vi "Update History Messages.vi"(8 "error in (no error)":errorcluster, 10 "Message":variant, 11 "Telegram Class in":refnum<class "Telegram Class.lvclass">) -> (0 "error out":errorcluster, 3 "Telegram Class out":refnum<class "Telegram Class.lvclass">)   [LabVIEW 2015, in "Telegram Library.lvlib" / "Telegram Class.lvclass"]
doc: "Created IvanLis by LabVIEW Portal\nProfile: http://labviewportal.org/memberlist.php?mode=viewprofile&u=987\neMail: IvanLisanov@gMail.com\nTelegram: https://t.me/IvanLis"
uses:
  Telegram Class.lvclass
  JSON Library/TypeDef/Message Text.ctl
  Telegram Class.lvclass/Telegram Class.ctl
  TypeDef/Message.ctl
  JSON Library/JSON Library.lvlib
  Telegram Library.lvlib
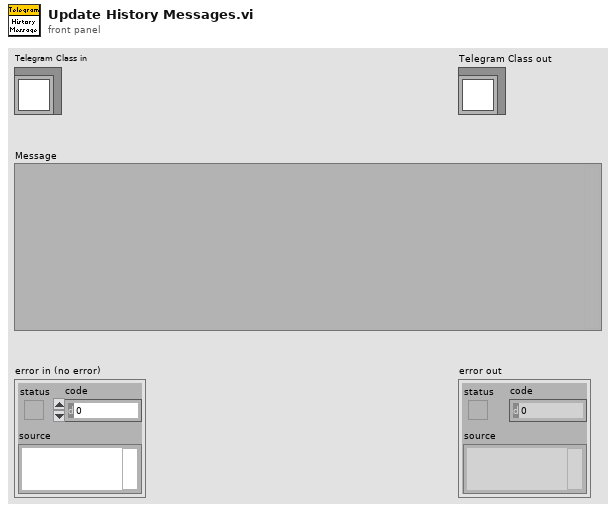
[diagram p1: front panel]
types:
  T1 = typedef "JSON Library.lvlib/Message Text.ctl" = cluster{"@type":string, "id":i64, "sender_id":cluster{"@type":string, "user_id":i64}, "chat_id":i64, "date":i64, "content":cluster{"@type":string, "text":cluster{"@type":string, "text":string}}}
  T2 = typedef "Telegram Library.lvlib/Message.ctl" = cluster{"id":i64, "chat_id":i64, "sender_user_id":i64, "date UTC":timestamp, "content_text":string}
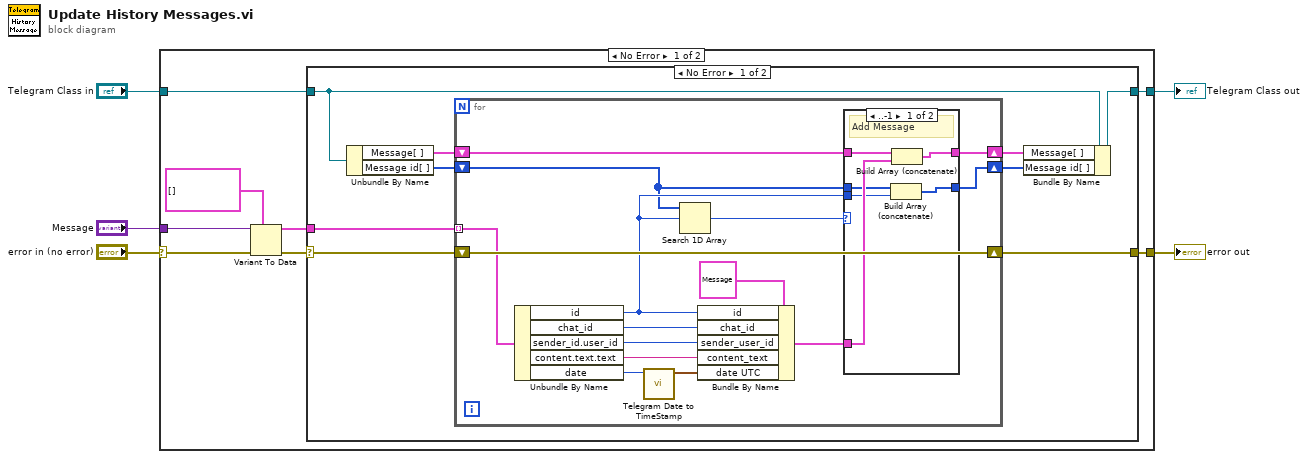
[diagram p0: block diagram]
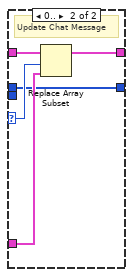
[diagram p2: hidden frame]
diagram:
  n1 = case shown="No Error" "error in (no error)" {
    selector: "error in (no error)" -> [w13 w52]
    tunnel: [w7 w52] -> w4
    tunnel: [w9 w51] -> w2
    tunnel: "Telegram Class in" -> [w10 w51]
    tunnel: "Message" -> [w11 _]
    frame No Error {
      n2 = Variant To Data(error in=w13, type=T1[] [] ("Array"), Variant=w11) -> (data=w6:T1[], error out=w8:errorcluster)
      n3 = case shown="No Error" w8 {
        selector: w8 -> [w22 w50]
        tunnel: w6 -> [w20 _]
        tunnel: [w21 w50] -> w7
        tunnel: w10 -> [w15 w49]
        tunnel: [w14 w49] -> w9
        frame No Error {
          n4 = Unbundle By Name(w15) -> ("Message[ ]"=w19:T2[], "Message id[ ]"=w18:i64[])
          n5 = for {
            shift-right: [w37] -> w21
            shift-left: w22 -> [w37]
            tunnel: w20 -> [w36] mode=indexing
            shift-right: [w24] -> w17
            shift-left: w19 -> [w26]
            shift-right: [w23] -> w16
            shift-left: w18 -> [w25]
            n6 = Unbundle By Name(w36) -> ("id"=w27:i64, "chat_id"=w28:i64, "sender_id.user_id"=w34:i64, "content.text.text"=w30:string, "date"=w33:i64)
            n7 = call "Telegram Date to TimeStamp.vi"("date"=w33) -> ("time stamp"=w32:timestamp)  [unwired: 10 in]
            n8 = Search 1D Array(1D array=w25, element=w27) -> (index of element=w31:i32)  [unwired: 1 in]
            n9 = Bundle By Name(cluster=T2 {"id"=0, "chat_id"=0, "sender_user_id"=0, "date UTC"=timestamp(0 s since 1904-01-01), "content_text"=""} ("Message"), "id"=w27, "chat_id"=w28, "sender_user_id"=w34, "content_text"=w30, "date UTC"=w32) -> (w29:T2)
            n10 = case shown="..-1" w31 {
              selector: w31 -> [_ w46]
              tunnel: w26 -> [w43 w48]
              tunnel: w29 -> [w42 w47]
              tunnel: [w41 w45] -> w24
              tunnel: w25 -> [w40 w44]
              tunnel: w27 -> [w39 _]
              tunnel: [w38 w44] -> w23
              frame ..-1 {
                # "Add Message"
                n11 = Build Array (concatenate)(w40, w39) -> (w38:i64[])
                n12 = Build Array (concatenate)(w43, w42) -> (w41:T2[])
              }
              frame 0.. {
                # "Update Chat Message"
                n13 = Replace Array Subset(array=w48, new element=w47, index=w46) -> (w45:T2[])
              }
            }
          }
          n14 = Bundle By Name(cluster=w15, "Message[ ]"=w17, "Message id[ ]"=w16) -> (w14:refnum<class "Telegram Class.lvclass">)
        }
        frame Error {
        }
      }
    }
    frame Error {
    }
  }
  "error out" <- w4
  "Telegram Class out" <- w2
